vi "array managment.vi"(0 "2D array in":dbl[][](array[numeric]), 1 "col sel":i32, 2 "cir num":i32, 3 "index":i32, 5 "subarray":dbl[](array[numeric])) -> (15 "2D array out":dbl[][](array[numeric]), 17 "1D array out":dbl[](array[numeric]))   [LabVIEW 2019]
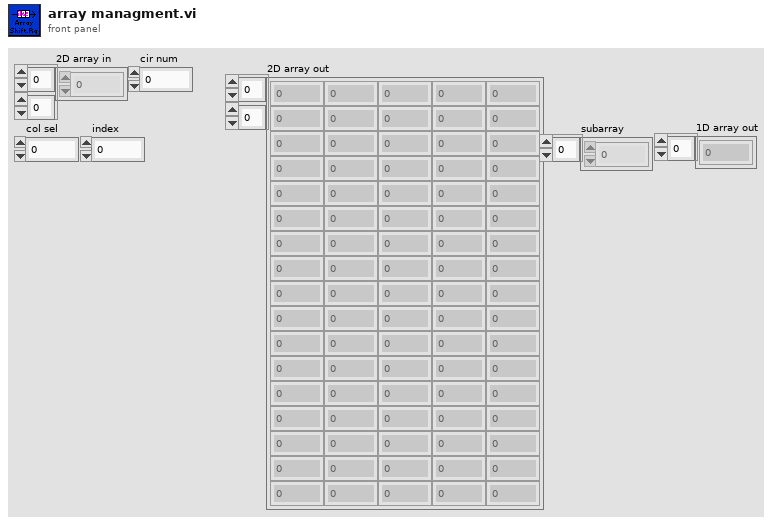
[diagram p1: front panel]
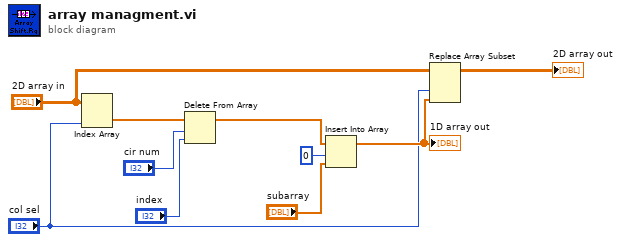
[diagram p0: block diagram]
diagram:
  n1 = Index Array "Index Array"(array="2D array in", index (col)="col sel") -> (element=w9:dbl[])  [unwired: 1 in]
  n2 = Delete From Array "Delete From Array"(array=w9, length="cir num", index="index") -> (array with subset deleted=w6:dbl[])  [unwired: 1 out]
  n3 = Insert Into Array "Insert Into Array"(array=w6, index=0, new element="subarray") -> (w5:dbl[])
  "1D array out" <- w5
  n4 = Replace Array Subset "Replace Array Subset"(array="2D array in", new element=w5, index (col)="col sel") -> (→"2D array out":dbl[][])  [unwired: 1 in]
